vi "Create SUBACK Packet.vi"(5 "SUBACK in":refnum<class "SUBACK.lvclass">, 8 "error in (no error)":errorcluster, 9 "Packet ID":u16 format="%04x", 11 "Return Codes":T1[](array[typedef])) -> (0 "error out":errorcluster, 2 "Bytes Stream":u8[](array[numeric]) format="%08b", 3 "SUBACK":refnum<class "SUBACK.lvclass">)   [LabVIEW 2013, in "MQTT_Control_Packets.lvlib" / "SUBACK.lvclass"]
uses:
  SUBACK.lvclass
  Subscription Success Code.ctl
  ControlPacket/QualityOfService -- enum.ctl
  ControlPacket/ControlPacket.lvclass/ControlPacket.ctl
  ControlPacket/ControlPacket.lvclass
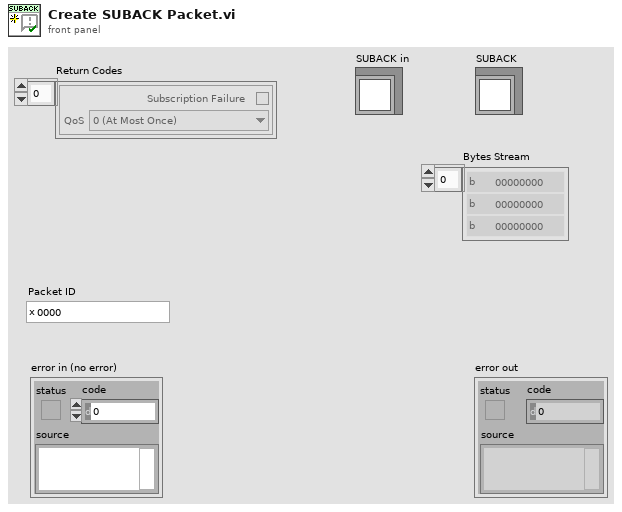
[diagram p1: front panel]
types:
  T1 = typedef "MQTT_Control_Packets.lvlib/SUBACK.lvclass/Subscription Success Code.ctl" = cluster{"Subscription Failure":bool, "QoS":T2}
  T2 = typedef "MQTT_Control_Packets.lvlib/ControlPacket.lvclass/QualityOfService -- enum.ctl" = enum16{"0 (At Most Once)", "1 (At Least Once)", "2 (Exactly Once)"}
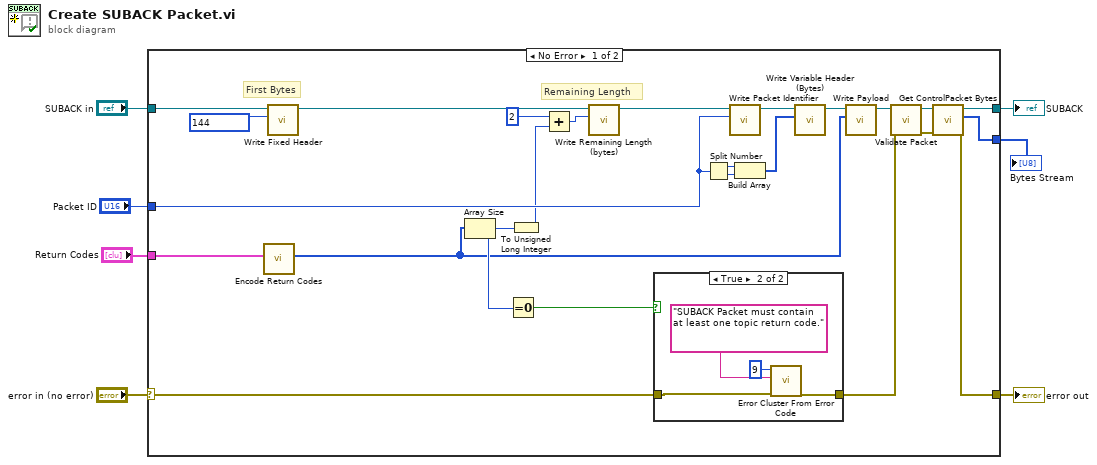
[diagram p0: block diagram]
diagram:
  n1 = case shown="No Error" "error in (no error)" {
    selector: "error in (no error)" -> [w18 w39]
    tunnel: [w11 w39] -> w4
    tunnel: [w9 w38] -> w3
    tunnel: "SUBACK in" -> [w32 w38]
    tunnel: "Packet ID" -> [w24 _]
    tunnel: "Return Codes" -> [w16 _]
    tunnel: [w10 _] -> w1
    frame No Error {
      # "Remaining Length"
      # "First Bytes"
      n2 = call "Encode Return Codes.vi"("Subscription Success"=w16) -> ("Return Codes"=w15:u8[])  [unwired: 10 in]
      n3 = call "Write Fixed Header.vi"("Fixed Header"=u8 144, "ControlPacket in"=w32) -> ("ControlPacket out"=w31:refnum<class "SUBACK.lvclass">)  [unwired: 9 in]
      n4 = Array Size(array=w15) -> (size(s)=w19:i32)
      n5 = Equal To 0?(x=w19) -> (x = 0?=w17:bool)
      n6 = To Unsigned Long Integer(number=w19) -> (unsigned 32bit integer=w20:u32)
      n7 = Add(x=u32 2 ("Remaining Length (bytes)"), y=w20) -> (x+y=w22:u32)
      n8 = call "Write Remaining Length (bytes).vi"("Remaining Length (bytes)"=w22, "ControlPacket in"=w31) -> ("ControlPacket out"=w27:refnum<class "SUBACK.lvclass">)  [unwired: 9 in]
      n9 = case shown="True" w17 {
        tunnel: w18 -> [w33 w36]
        tunnel: [w33 w37] -> w13
        frame False {
        }
        frame True {
          n10 = call <vilib>:"Error Cluster From Error Code.vi"("error in (no error)"=w36, "error message (\"\")"="SUBACK Packet must contain at least one topic return code.", "error code (0)"=9) -> ("error out"=w37:errorcluster)  [unwired: 6 in]
        }
      }
      n11 = Split Number(x=w24) -> (hi(x)=w30:u8, lo(x)=w29:u8)
      n12 = call "Write Packet Identifier.vi"("Packet Identifier"=w24, "ControlPacket in"=w27) -> ("ControlPacket out"=w26:refnum<class "SUBACK.lvclass">)  [unwired: 9 in]
      n13 = Build Array(w30, w29) -> (w28:u8[])
      n14 = call "Write Variable Header (Bytes).vi"("Variable Header (Bytes)"=w28, "ControlPacket in"=w26) -> ("ControlPacket out"=w21:refnum<class "SUBACK.lvclass">)  [unwired: 9 in]
      n15 = call "Write Payload.vi"("Payload"=w15, "ControlPacket in"=w21) -> ("ControlPacket out"=w14:refnum<class "SUBACK.lvclass">)  [unwired: 9 in]
      n16 = call "Validate Packet.vi"("error in (no error)"=w13, "ControlPacket in"=w14) -> ("error out"=w12:errorcluster, "ControlPacket out"=w8:refnum<class "SUBACK.lvclass">)  [unwired: 8 in]
      n17 = call "Get ControlPacket Bytes.vi"("error in (no error)"=w12, "ControlPacket"=w8) -> ("error out"=w11:errorcluster, "Bytes Stream"=w10:u8[], "ControlPacket dup"=w9:refnum<class "SUBACK.lvclass">)  [unwired: 6 in, 1 out]
    }
    frame Error {
    }
  }
  "error out" <- w4
  "SUBACK" <- w3
  "Bytes Stream" <- w1
